vi "SplineHelp_getCubicSplinesFromControlVectors.vi"(9 "endCtrlVector":T3, 10 "InternalWaypoints":T4[](array[typedef]) {"Y" format="%14.3f"; "X" format="%14.3f"}, 11 "startCtrlVector":T3) -> (0 "error out":errorcluster, 3 "splines":T1[](array[typedef]), 4 "y final":dbl[][](array[numeric]), 5 "x final":dbl[][](array[numeric]), 6 "y init":dbl[][](array[numeric]), 7 "x init":dbl[][](array[numeric]))   [LabVIEW 2019, in "Trajectory_Library.lvlib"]
doc: "Returns a set of cubic splines corresponding to the provided control vectors. The user is free to set the direction of the start and end point. The directions for the middle waypoints are determined automatically to ensure continuous curvature throughout the path.\n\nParameters: \n - startCtrlVector - The starting control vector.\n - waypoints - The middle waypoints. This can be left blank if you only wish to create a path with two waypoints.\n - endCtrlVector - The ending control vector.\n\nReturns:\n - A vector of cubic hermite splines that interpolate through the provided waypoints and control vectors.\n - Error Out - Output error cluster\n - X init - For diagnostics only (these may be deleted in the future)\n - X final - For diagnostics only (these may be deleted in the future)\n - Y init - For diagnostics only (these may be deleted in the future)\n - Y final - For diagnostics only (these may be deleted in the future)"
uses:
  Trajectory_Library.lvlib
  SPLINE_CTRL_VECTOR.ctl
  TRANSLATION2D.ctl
  SPLINE.ctl
  <vilib>/Analysis/Matrix/Datatypes/RealMatrix.ctl
  <vilib>/Analysis/Matrix/NI_Matrix.lvlib
panel:
  # "for\ndebug!"
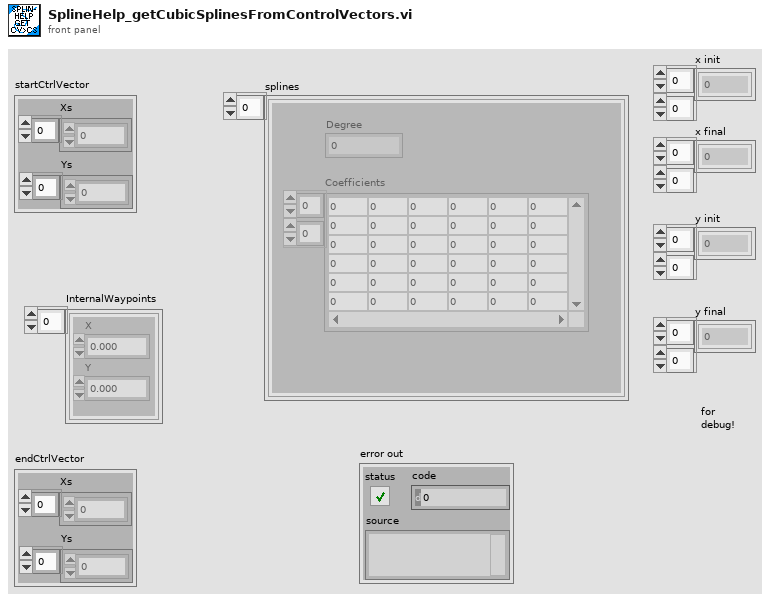
[diagram p1: front panel]
types:
  T1 = typedef "Trajectory_Library.lvlib/SPLINE.ctl" = cluster{"Degree":i32, "Coefficients":T2}
  T2 = typedef "NI_Matrix.lvlib/RealMatrix.ctl" = dbl[][]
  T3 = typedef "Trajectory_Library.lvlib/SPLINE_CTRL_VECTOR.ctl" = cluster{"Xs":dbl[], "Ys":dbl[]}
  T4 = typedef "Trajectory_Library.lvlib/TRANSLATION2D.ctl" = cluster{"X":dbl, "Y":dbl}
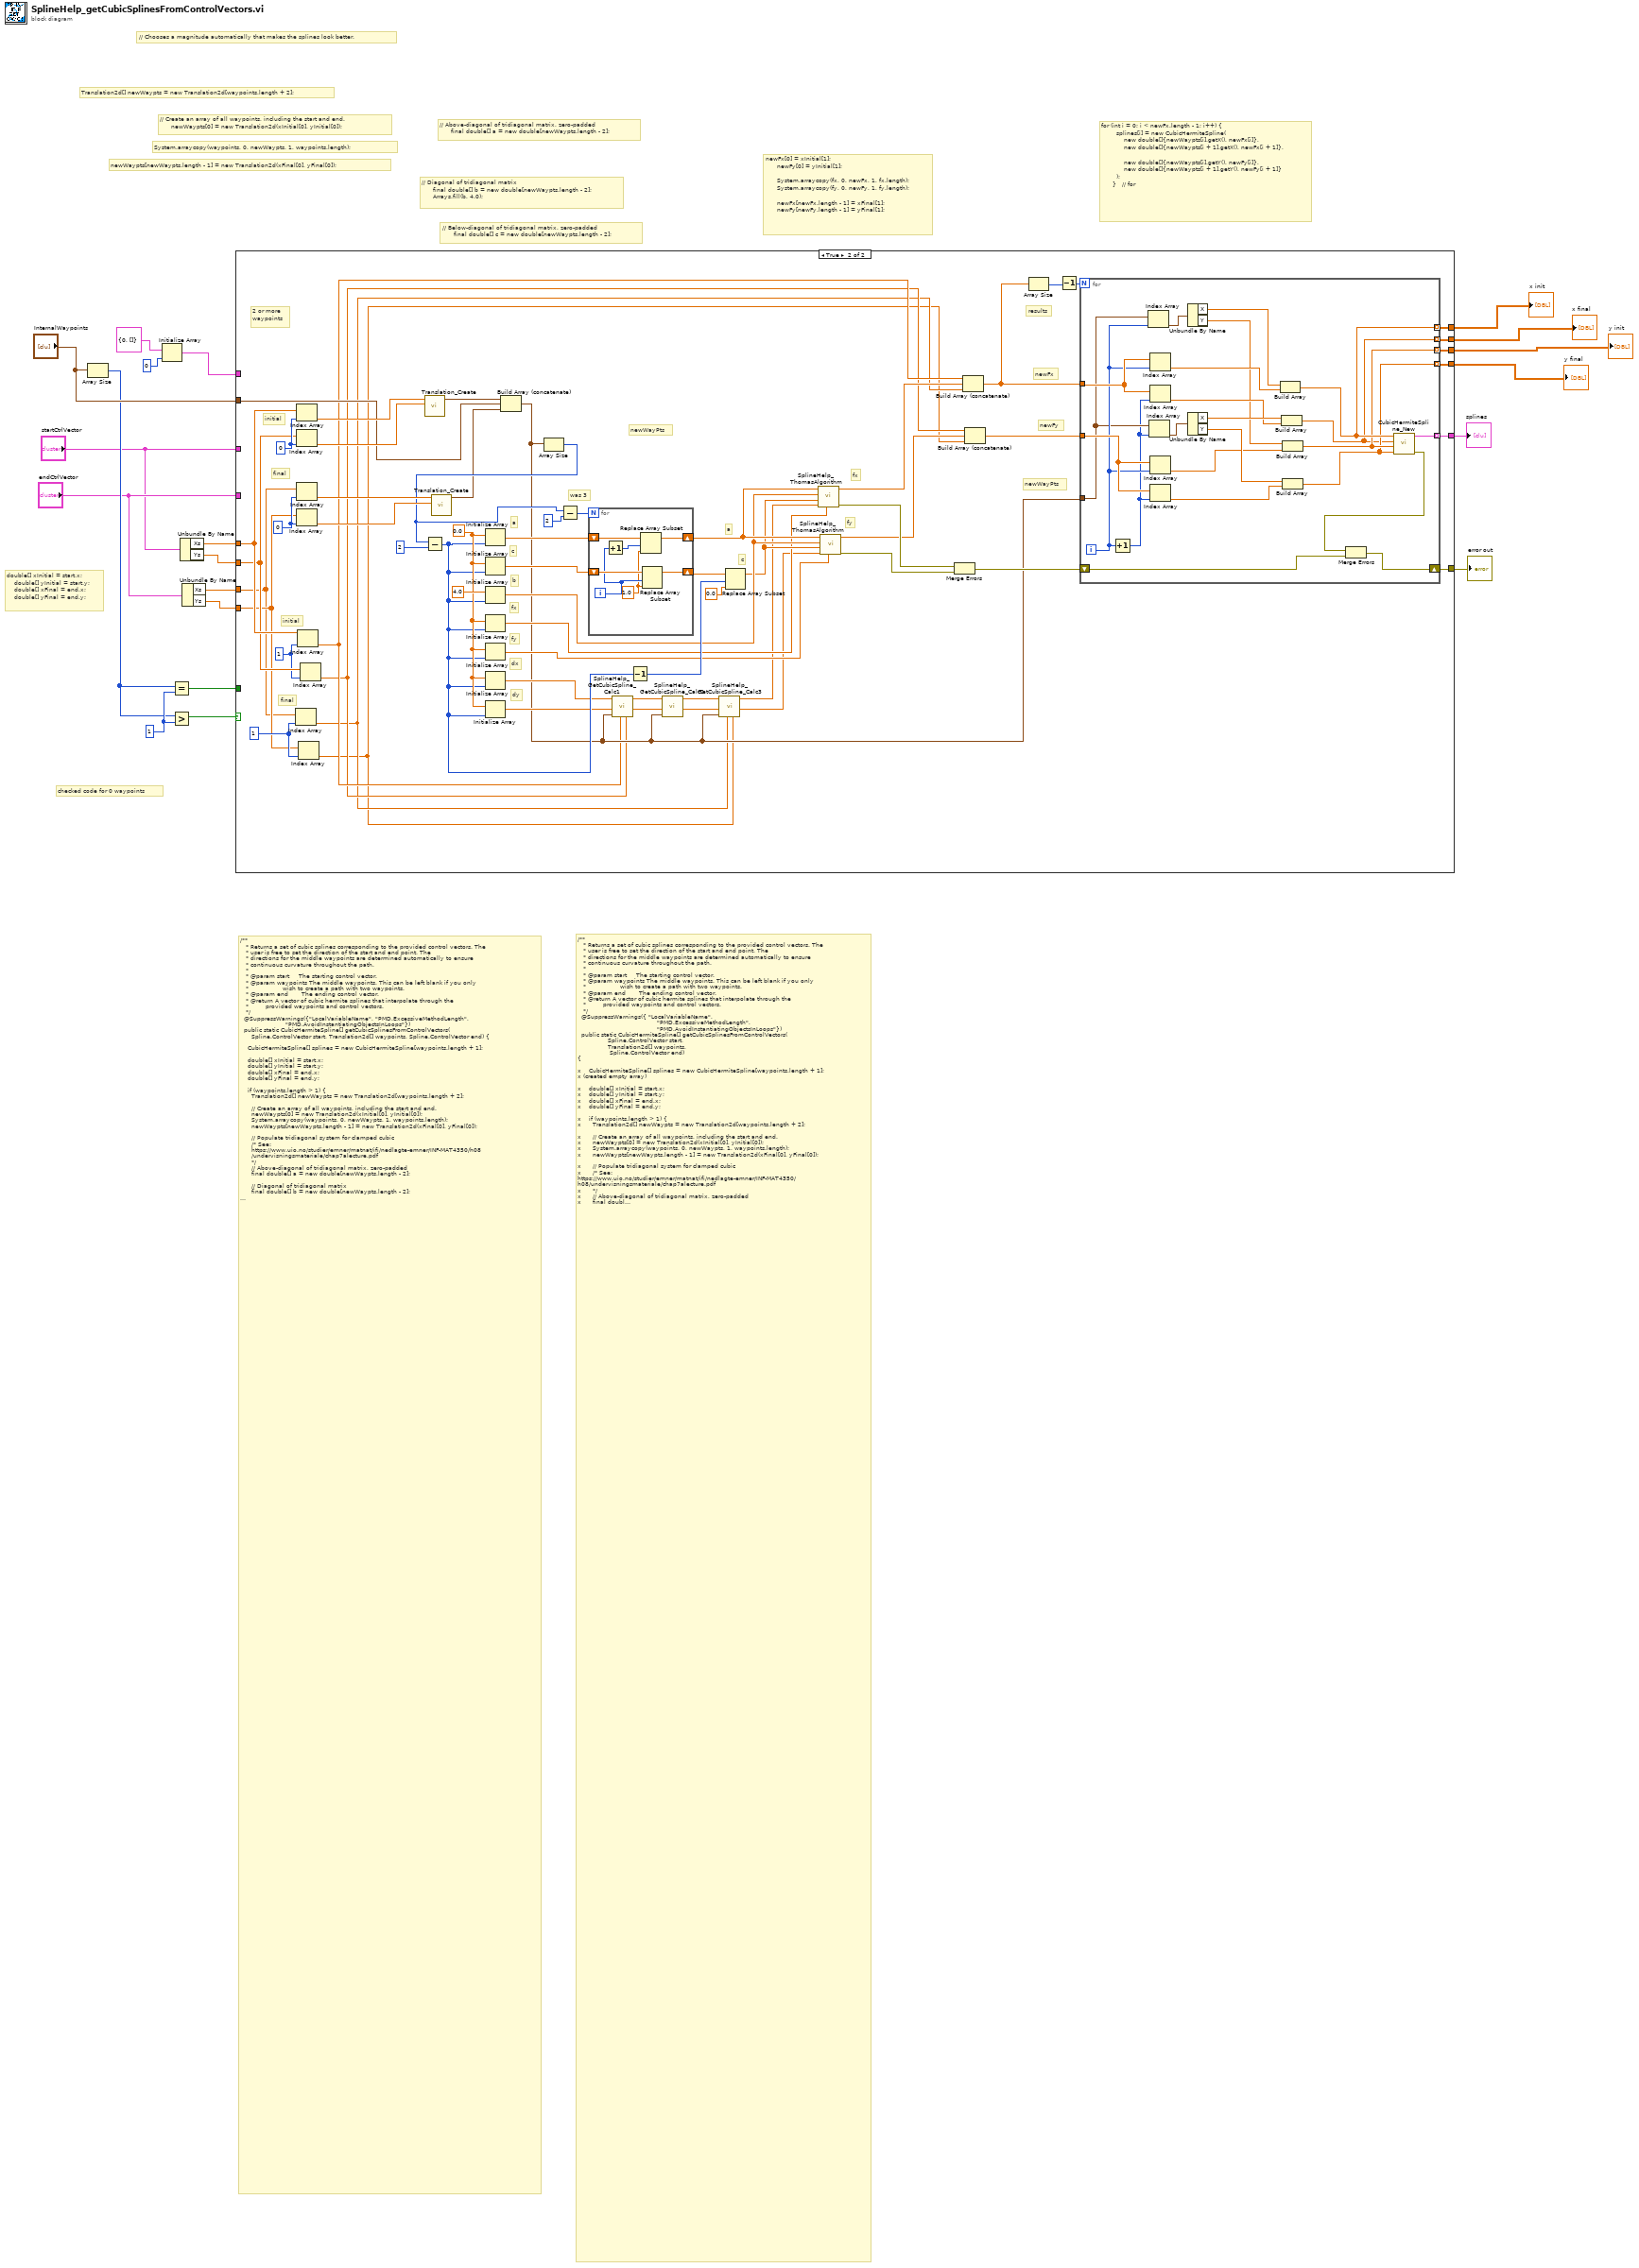
[diagram p0: block diagram]
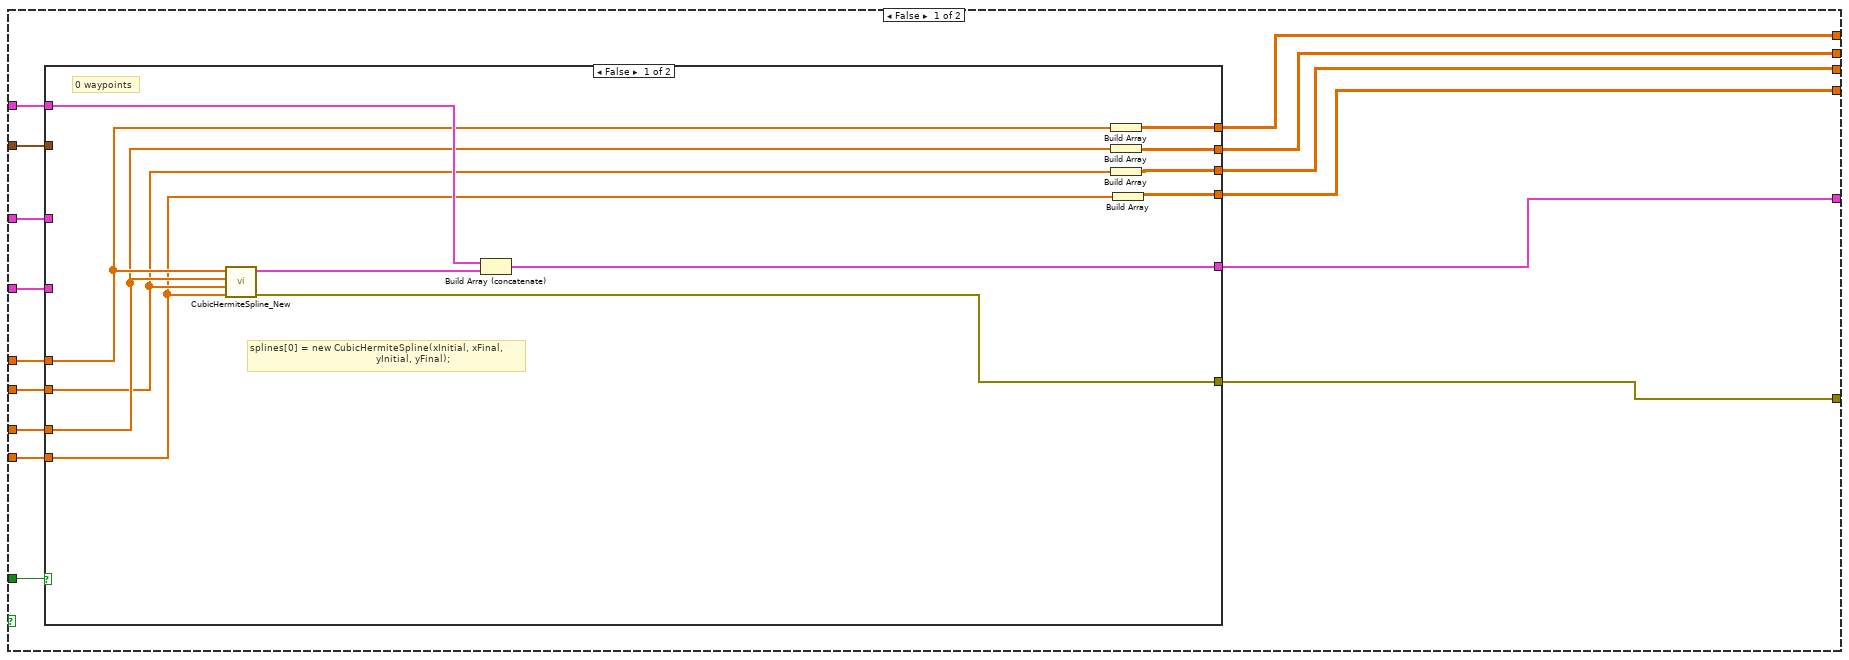
[diagram p2: hidden frame]
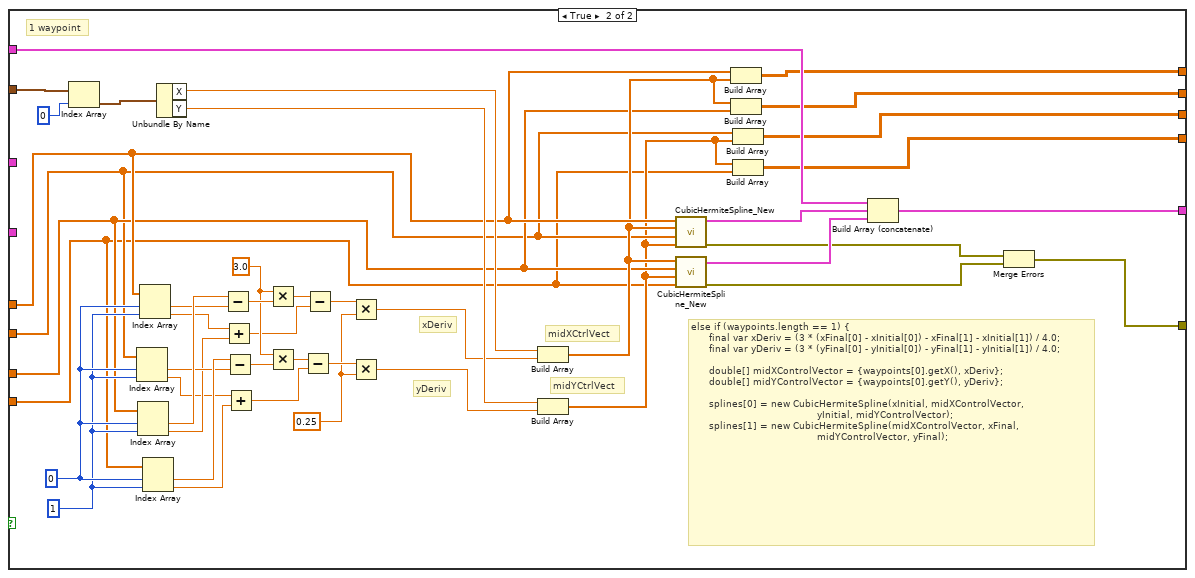
[diagram p3: hidden frame]
diagram:
  w18 = 1 ("y")
  # "for (int i = 0; i < newFx.length - 1; i++) {\n        splines[i] = new CubicHermiteSpline(\n            new double[]{newWaypts[i].getX(), newFx[i]},\n            new double[]{newWaypts[i + 1].getX(), newFx[i + 1]},\n\n            new double[]{newWaypts[i].getY(), newFy[i]},\n            new double[]{newWaypts[i + 1].getY(), newFy[i + 1]}\n        );\n      }   // for"
  # "/**\n   * Returns a set of cubic splines corresponding to the provided control vectors. The\n   * user is free to set the direction of the start and end point. The\n   * directions for the middle waypoints are determined automatically to ensure\n   * continuous curvature throughout the path.\n   *\n   * @param start     The starting control vector.\n   * @param waypoints The middle waypoints. This can be left blank if you only\n   *                  wish to create a path with two waypoints.\n   * @param end       The ending control vector.\n   * @return A vector of cubic hermite splines that interpolate through the\n   *         provided waypoints and control vectors.\n   */\n  @SuppressWarnings({ \"LocalVariableName\", \n                                          \"PMD.ExcessiveMethodLength\",\n                                          \"PMD.AvoidInstantiatingObjectsInLoops\"})\n  public static CubicHermiteSpline[] getCubicSplinesFromControlVectors(\n                Spline.ControlVector start, \n                Translation2d[] waypoints, \n                 Spline.ControlVector end) \n{\n\nx    CubicHermiteSpline[] splines = new CubicHermiteSpline[waypoints.length + 1];\nx (created empty array)\n\nx    double[] xInitial = start.x;\nx    double[] yInitial = start.y;\nx    double[] xFinal = end.x;\nx    double[] yFinal = end.y;\n\nx    if (waypoints.length > 1) {\nx      Translation2d[] newWaypts = new Translation2d[waypoints.length + 2];\n\nx      // Create an array of all waypoints, including the start and end.\nx      newWaypts[0] = new Translation2d(xInitial[0], yInitial[0]);\nx      System.arraycopy(waypoints, 0, newWaypts, 1, waypoints.length);\nx      newWaypts[newWaypts.length - 1] = new Translation2d(xFinal[0], yFinal[0]);\n\nx      // Populate tridiagonal system for clamped cubic\nx      /* See:      \nhttps://www.uio.no/studier/emner/matnat/ifi/nedlagte-emner/INF-MAT4350/\nh08/undervisningsmateriale/chap7alecture.pdf\nx      */\nx      // Above-diagonal of tridiagonal matrix, zero-padded\nx      final double[] a = new double[newWaypts.length - 2];\n\nx      // Diagonal of tridiagonal matrix\nx      final double[] b = new double[newWaypts.length - 2];\nx      Arrays.fill(b, 4.0);\n\nx      // Below-diagonal of tridiagonal matrix, zero-padded\nx      final double[] c = new double[newWaypts.length - 2];\n\nx      // rhs vectors\nx      final double[] dx = new double[newWaypts.length - 2];\nx      final double[] dy = new double[newWaypts.length - 2];\n\nx      // solution vectors\nx      final double[] fx = new double[newWaypts.length - 2];\nx      final double[] fy = new double[newWaypts.length - 2];\n\n      // populate above-diagonal and below-diagonal vectors\nx      a[0] = 0.0;\nx      for (int i = 0; i < newWaypts.length - 3; i++) {\nx        a[i + 1] = 1;\nx        c[i] = 1;\nx      }   //for\nx      c[c.length - 1] = 0.0;\n\nx SUBVI - CALC 1\nx      // populate rhs vectors\nx      dx[0] = 3 * (newWaypts[2].getX() - newWaypts[0].getX()) - xInitial[1];\nx      dy[0] = 3 * (newWaypts[2].getY() - newWaypts[0].getY()) - yInitial[1];\n\nx SUBVI - CALC 2\nx      if (newWaypts.length > 4)  { \nx        for (int i = 1; i <= newWaypts.length - 4; i++) {\nx          dx[i] = 3 * (newWaypts[i + 1].getX() - newWaypts[i - 1].getX());\nx          dy[i] = 3 * (newWaypts[i + 1].getY() - newWaypts[i - 1].getY());\nx        }  // for\nx      } // > 4\n\nx SUBVI - CALC 3\nx      dx[dx.length - 1] = 3 * (newWaypts[newWaypts.length - 1].getX()\nx          - newWaypts[newWaypts.length - 3].getX()) - xFinal[1];\nx      dy[dy.length - 1] = 3 * (newWaypts[newWaypts.length - 1].getY()\nx          - newWaypts[newWaypts.length - 3].getY()) - yFinal[1];\n\nx      // Compute solution to tridiagonal system\nx      thomasAlgorithm(a, b, c, dx, fx);\nx      thomasAlgorithm(a, b, c, dy, fy);\n\nx      double[] newFx = new double[fx.length + 2];\nx      double[] newFy = new double[fy.length + 2];\n\nx      newFx[0] = xInitial[1];\nx      newFy[0] = yInitial[1];\nx      System.arraycopy(fx, 0, newFx, 1, fx.length);\nx      System.arraycopy(fy, 0, newFy, 1, fy.length);\nx      newFx[newFx.length - 1] = xFinal[1];\nx      newFy[newFy.length - 1] = yFinal[1];\n\n      for (int i = 0; i < newFx.length - 1; i++) {\n        splines[i] = new CubicHermiteSpline(\n            new double[]{newWaypts[i].getX(), newFx[i]},\n            new double[]{newWaypts[i + 1].getX(), newFx[i + 1]},\n            new double[]{newWaypts[i].getY(), newFy[i]},\n            new double[]{newWaypts[i + 1].getY(), newFy[i + 1]}\n        );\n      }   // for\n    } else if (waypoints.length == 1) {\n      final var xDeriv = (3 * (xFinal[0]\n          - xInitial[0])\n          - xFinal[1] - xInitial[1])\n          / 4.0;\n      final var yDeriv = (3 * (yFinal[0]\n          - yInitial[0])\n          - yFinal[1] - yInitial[1])\n          / 4.0;\n\n      double[] midXControlVector = {waypoints[0].getX(), xDeriv};\n      double[] midYControlVector = {waypoints[0].getY(), yDeriv};\n\n      splines[0] = new CubicHermiteSpline(xInitial, midXControlVector,\n                                          yInitial, midYControlVector);\n      splines[1] = new CubicHermiteSpline(midXControlVector, xFinal,\n                                          midYControlVector, yFinal);\n    } else {\n      splines[0] = new CubicHermiteSpline(xInitial, xFinal,\n                                          yInitial, yFinal);\n    }\n    return splines;\n  }"
  # "// Below-diagonal of tridiagonal matrix, zero-padded\n      final double[] c = new double[newWaypts.length - 2];"
  # "// Diagonal of tridiagonal matrix\n      final double[] b = new double[newWaypts.length - 2];\n      Arrays.fill(b, 4.0);"
  # "// Above-diagonal of tridiagonal matrix, zero-padded\n      final double[] a = new double[newWaypts.length - 2];"
  # "newWaypts[newWaypts.length - 1] = new Translation2d(xFinal[0], yFinal[0]);"
  # "System.arraycopy(waypoints, 0, newWaypts, 1, waypoints.length);"
  # "// Create an array of all waypoints, including the start and end.\n      newWaypts[0] = new Translation2d(xInitial[0], yInitial[0]);"
  # "Translation2d[] newWaypts = new Translation2d[waypoints.length + 2];"
  # "checked code for 0 waypoints"
  # "double[] xInitial = start.x;\n    double[] yInitial = start.y;\n    double[] xFinal = end.x;\n    double[] yFinal = end.y;"
  # "newFx[0] = xInitial[1];\n      newFy[0] = yInitial[1];\n\n      System.arraycopy(fx, 0, newFx, 1, fx.length);\n      System.arraycopy(fy, 0, newFy, 1, fy.length);\n\n      newFx[newFx.length - 1] = xFinal[1];\n      newFy[newFy.length - 1] = yFinal[1];"
  # "/**\n   * Returns a set of cubic splines corresponding to the provided control vectors. The\n   * user is free to set the direction of the start and end point. The\n   * directions for the middle waypoints are determined automatically to ensure\n   * continuous curvature throughout the path.\n   *\n   * @param start     The starting control vector.\n   * @param waypoints The middle waypoints. This can be left blank if you only\n   *                  wish to create a path with two waypoints.\n   * @param end       The ending control vector.\n   * @return A vector of cubic hermite splines that interpolate through the\n   *         provided waypoints and control vectors.\n   */\n  @SuppressWarnings({\"LocalVariableName\", \"PMD.ExcessiveMethodLength\",\n                        \"PMD.AvoidInstantiatingObjectsInLoops\"})\n  public static CubicHermiteSpline[] getCubicSplinesFromControlVectors(\n      Spline.ControlVector start, Translation2d[] waypoints, Spline.ControlVector end) {\n\n    CubicHermiteSpline[] splines = new CubicHermiteSpline[waypoints.length + 1];\n\n    double[] xInitial = start.x;\n    double[] yInitial = start.y;\n    double[] xFinal = end.x;\n    double[] yFinal = end.y;\n\n    if (waypoints.length > 1) {\n      Translation2d[] newWaypts = new Translation2d[waypoints.length + 2];\n\n      // Create an array of all waypoints, including the start and end.\n      newWaypts[0] = new Translation2d(xInitial[0], yInitial[0]);\n      System.arraycopy(waypoints, 0, newWaypts, 1, waypoints.length);\n      newWaypts[newWaypts.length - 1] = new Translation2d(xFinal[0], yFinal[0]);\n\n      // Populate tridiagonal system for clamped cubic\n      /* See:\n      https://www.uio.no/studier/emner/matnat/ifi/nedlagte-emner/INF-MAT4350/h08\n      /undervisningsmateriale/chap7alecture.pdf\n      */\n      // Above-diagonal of tridiagonal matrix, zero-padded\n      final double[] a = new double[newWaypts.length - 2];\n\n      // Diagonal of tridiagonal matrix\n      final double[] b = new double[newWaypts.length - 2];\n      Arrays.fill(b, 4.0);\n\n      // Below-diagonal of tridiagonal matrix, zero-padded\n      final double[] c = new double[newWaypts.length - 2];\n\n      // rhs vectors\n      final double[] dx = new double[newWaypts.length - 2];\n      final double[] dy = new double[newWaypts.length - 2];\n\n      // solution vectors\n      final double[] fx = new double[newWaypts.length - 2];\n      final double[] fy = new double[newWaypts.length - 2];\n\n      // populate above-diagonal and below-diagonal vectors\n      a[0] = 0.0;\n      for (int i = 0; i < newWaypts.length - 3; i++) {\n        a[i + 1] = 1;\n        c[i] = 1;\n      }\n      c[c.length - 1] = 0.0;\n\n      // populate rhs vectors\n      dx[0] = 3 * (newWaypts[2].getX() - newWaypts[0].getX()) - xInitial[1];\n      dy[0] = 3 * (newWaypts[2].getY() - newWaypts[0].getY()) - yInitial[1];\n\n      if (newWaypts.length > 4) {\n        for (int i = 1; i <= newWaypts.length - 4; i++) {\n          dx[i] = 3 * (newWaypts[i + 1].getX() - newWaypts[i - 1].getX());\n          dy[i] = 3 * (newWaypts[i + 1].getY() - newWaypts[i - 1].getY());\n        }\n      }\n\n      dx[dx.length - 1] = 3 * (newWaypts[newWaypts.length - 1].getX()\n          - newWaypts[newWaypts.length - 3].getX()) - xFinal[1];\n      dy[dy.length - 1] = 3 * (newWaypts[newWaypts.length - 1].getY()\n          - newWaypts[newWaypts.length - 3].getY()) - yFinal[1];\n\n      // Compute solution to tridiagonal system\n      thomasAlgorithm(a, b, c, dx, fx);\n      thomasAlgorithm(a, b, c, dy, fy);\n\n      double[] newFx = new double[fx.length + 2];\n      double[] newFy = new double[fy.length + 2];\n\n      newFx[0] = xInitial[1];\n      newFy[0] = yInitial[1];\n      System.arraycopy(fx, 0, newFx, 1, fx.length);\n      System.arraycopy(fy, 0, newFy, 1, fy.length);\n      newFx[newFx.length - 1] = xFinal[1];\n      newFy[newFy.length - 1] = yFinal[1];\n\n      for (int i = 0; i < newFx.length - 1; i++) {\n        splines[i] = new CubicHermiteSpline(\n            new double[]{newWaypts[i].getX(), newFx[i]},\n            new double[]{newWaypts[i + 1].getX(), newFx[i + 1]},\n            new double[]{newWaypts[i].getY(), newFy[i]},\n            new double[]{newWaypts[i + 1].getY(), newFy[i + 1]}\n        );\n      }\n    } else if (waypoints.length == 1) {\n      final var xDeriv = (3 * (xFinal[0]\n          - xInitial[0])\n          - xFinal[1] - xInitial[1])\n          / 4.0;\n      final var yDeriv = (3 * (yFinal[0]\n          - yInitial[0])\n          - yFinal[1] - yInitial[1])\n          / 4.0;\n\n      double[] midXControlVector = {waypoints[0].getX(), xDeriv};\n      double[] midYControlVector = {waypoints[0].getY(), yDeriv};\n\n      splines[0] = new CubicHermiteSpline(xInitial, midXControlVector,\n                                          yInitial, midYControlVector);\n      splines[1] = new CubicHermiteSpline(midXControlVector, xFinal,\n                                          midYControlVector, yFinal);\n    } else {\n      splines[0] = new CubicHermiteSpline(xInitial, xFinal,\n                                          yInitial, yFinal);\n    }\n    return splines;\n  }"
  # "// Chooses a magnitude automatically that makes the splines look better."
  n1 = Array Size(array="InternalWaypoints") -> (size(s)=w12:i32)
  n2 = Initialize Array(T1 {"Degree"=0, "Coefficients"=[]} ("SPLINE"), 0 ("dimension size")) -> (w14:T1[])
  n3 = Equal?(x=w12, y=w18) -> (x = y?=w17:bool)
  n4 = Greater?(x=w12, y=w18) -> (0:w19:bool)
  n5 = Unbundle By Name("startCtrlVector") -> ("Xs"=w9:dbl[], "Ys"=w8:dbl[])
  n6 = Unbundle By Name("endCtrlVector") -> ("Xs"=w7:dbl[], "Ys"=w6:dbl[])
  n7 = case shown="True" w19 {
    tunnel: w17 -> [w35 _]
    tunnel: w14 -> [w34 _]
    tunnel: [w33 w130] -> w16
    tunnel: [w32 w123] -> w15
    tunnel: "startCtrlVector" -> [w31 _]
    tunnel: "endCtrlVector" -> [w30 _]
    tunnel: "InternalWaypoints" -> [w29 w106]
    tunnel: w9 -> [w28 w139]
    tunnel: w8 -> [w27 w138]
    tunnel: w7 -> [w26 w122]
    tunnel: w6 -> [w25 w128]
    tunnel: [w21 w95] -> w1
    tunnel: [w22 w94] -> w2
    tunnel: [w23 w93] -> w3
    tunnel: [w24 w92] -> w4
    frame False {
      n8 = case shown="False" w35 {
        tunnel: w34 -> [w47 w84]
        tunnel: [w46 w83] -> w33
        tunnel: [w44 w78] -> w32
        tunnel: w31 -> [_ _]
        tunnel: w30 -> [_ _]
        tunnel: w29 -> [_ w90]
        tunnel: w28 -> [w39 w57]
        tunnel: w27 -> [w37 w54]
        tunnel: w26 -> [w38 w55]
        tunnel: w25 -> [w36 w52]
        tunnel: [w43 w51] -> w24
        tunnel: [w42 w50] -> w23
        tunnel: [w41 w49] -> w22
        tunnel: [w40 w48] -> w21
        frame False {
          # "splines[0] = new CubicHermiteSpline(xInitial, xFinal,\n                                          yInitial, yFinal);"
          # "0 waypoints"
          n9 = call "CubicHermiteSpline_New.vi"("yFinalCtrlVector"=w36, "yInitialCtrlVector"=w37, "xFinalCtrlVector"=w38, "XInitialCtrlVector"=w39) -> ("error out"=w44:errorcluster, "CubicHermiteSpline"=w45:T1)  [unwired: 6 in]
          n10 = Build Array (concatenate)(w47, w45) -> (w46:T1[])
          n11 = Build Array(w39) -> (w43:dbl[][])
          n12 = Build Array(w38) -> (w42:dbl[][])
          n13 = Build Array(w37) -> (w41:dbl[][])
          n14 = Build Array(w36) -> (w40:dbl[][])
        }
        frame True {
          w60 = 0.25 ("y")
          w71 = 3.0 ("x")
          w85 = 1 ("index")
          w86 = 0 ("index")
          # "yDeriv"
          # "xDeriv"
          # "midYCtrlVect"
          # "midXCtrlVect"
          # "else if (waypoints.length == 1) {\n      final var xDeriv = (3 * (xFinal[0] - xInitial[0]) - xFinal[1] - xInitial[1]) / 4.0;\n      final var yDeriv = (3 * (yFinal[0] - yInitial[0]) - yFinal[1] - yInitial[1]) / 4.0;\n\n      double[] midXControlVector = {waypoints[0].getX(), xDeriv};\n      double[] midYControlVector = {waypoints[0].getY(), yDeriv};\n\n      splines[0] = new CubicHermiteSpline(xInitial, midXControlVector,\n                                          yInitial, midYControlVector);\n      splines[1] = new CubicHermiteSpline(midXControlVector, xFinal,\n                                          midYControlVector, yFinal);"
          # "1 waypoint"
          n15 = Index Array(array=w90, index=0) -> (element=w89:T4)
          n16 = Index Array(array=w54, index #1=w86, index #2=w85) -> (element #1=w74:dbl, element #2=w66:dbl)
          n17 = Index Array(array=w55, index #1=w86, index #2=w85) -> (element #1=w77:dbl, element #2=w70:dbl)
          n18 = Index Array(array=w57, index #1=w86, index #2=w85) -> (element #1=w76:dbl, element #2=w69:dbl)
          n19 = Index Array(array=w52, index #1=w86, index #2=w85) -> (element #1=w75:dbl, element #2=w65:dbl)
          n20 = Unbundle By Name(w89) -> ("X"=w88:dbl, "Y"=w87:dbl)
          n21 = Subtract(x=w77, y=w76) -> (x-y=w73:dbl)
          n22 = Add(x=w69, y=w70) -> (x+y=w67:dbl)
          n23 = Subtract(x=w75, y=w74) -> (x-y=w72:dbl)
          n24 = Add(x=w66, y=w65) -> (x+y=w63:dbl)
          n25 = Multiply(x=w71, y=w73) -> (x*y=w68:dbl)
          n26 = Multiply(x=w71, y=w72) -> (x*y=w64:dbl)
          n27 = Subtract(x=w64, y=w63) -> (x-y=w61:dbl)
          n28 = Subtract(x=w68, y=w67) -> (x-y=w62:dbl)
          n29 = Multiply(x=w62, y=w60) -> (x*y=w59:dbl)
          n30 = Multiply(x=w61, y=w60) -> (x*y=w58:dbl)
          n31 = Build Array(w88, w59) -> (w56:dbl[])
          n32 = Build Array(w87, w58) -> (w53:dbl[])
          n33 = call "CubicHermiteSpline_New.vi"("yFinalCtrlVector"=w53, "yInitialCtrlVector"=w54, "xFinalCtrlVector"=w56, "XInitialCtrlVector"=w57) -> ("error out"=w80:errorcluster, "CubicHermiteSpline"=w82:T1)  [unwired: 6 in]
          n34 = call "CubicHermiteSpline_New.vi"("yFinalCtrlVector"=w52, "yInitialCtrlVector"=w53, "xFinalCtrlVector"=w55, "XInitialCtrlVector"=w56) -> ("error out"=w79:errorcluster, "CubicHermiteSpline"=w81:T1)  [unwired: 6 in]
          n35 = Build Array(w57, w56) -> (w51:dbl[][])
          n36 = Build Array(w56, w55) -> (w50:dbl[][])
          n37 = Build Array(w54, w53) -> (w49:dbl[][])
          n38 = Build Array(w53, w52) -> (w48:dbl[][])
          n39 = Build Array (concatenate)(w84, w82, w81) -> (w83:T1[])
          n40 = Merge Errors(w80, w79) -> (w78:errorcluster)
        }
      }
    }
    frame True {
      w129 = 1 ("index")
      w137 = 1 ("index")
      w134 = 0.0
      w148 = 0 ("index")
      w151 = 0 ("index")
      # "was 3"
      # "newWayPts"
      # "newFy"
      # "newFx"
      # "2 or more\nwaypoints"
      # "results"
      # "initial"
      # "final"
      # "final"
      # "initial"
      # "fy"
      # "fx"
      # "c"
      # "a"
      # "dy"
      # "dx"
      # "fy"
      # "fx"
      # "b"
      # "c"
      # "a"
      # "newWayPts"
      n41 = Index Array(array=w122, index=w129) -> (element=w100:dbl)
      n42 = Index Array(array=w138, index=w151) -> (element=w149:dbl)
      n43 = Index Array(array=w128, index=w148) -> (element=w146:dbl)
      n44 = Index Array(array=w139, index=w151) -> (element=w150:dbl)
      n45 = Index Array(array=w122, index=w148) -> (element=w147:dbl)
      n46 = Index Array(array=w139, index=w137) -> (element=w102:dbl)
      n47 = Index Array(array=w128, index=w129) -> (element=w99:dbl)
      n48 = Index Array(array=w138, index=w137) -> (element=w101:dbl)
      n49 = call "Translation_Create.vi"("Y"=w149, "X"=w150) -> ("TRANSLATION"=w108:T4)  [unwired: 9 in]
      n50 = call "Translation_Create.vi"("Y"=w146, "X"=w147) -> ("TRANSLATION"=w107:T4)  [unwired: 9 in]
      n51 = Build Array (concatenate)(w108, w106, w107) -> (w105:T4[])
      n52 = Array Size(array=w105) -> (size(s)=w118:i32)
      n53 = Subtract(x=w118, y=2) -> (x-y=w117:i32)
      n54 = Initialize Array(w134, w117) -> (w145:dbl[])
      n55 = Initialize Array(w134, w117) -> (w136:dbl[])
      n56 = Initialize Array(4.0, w117) -> (w132:dbl[])
      n57 = Initialize Array(w134, w117) -> (w120:dbl[])
      n58 = Initialize Array(w134, w117) -> (w127:dbl[])
      n59 = Initialize Array(w134, w117) -> (w115:dbl[])
      n60 = Initialize Array(w134, w117) -> (w114:dbl[])
      n61 = Subtract(x=w118, y=2) -> (x-y=w144:i32)
      n62 = for {
        N: w144 -> [_]
        shift-right: [w175] -> w133
        shift-left: w145 -> [w181]
        shift-right: [w176] -> w141
        shift-left: w136 -> [w180]
        i -> [w178]
        w177 = 1.0 ("new element/subarray")
        n63 = Increment(x=w178) -> (x+1=w179:i32)
        n64 = Replace Array Subset(array=w181, new element=w177, index=w179) -> (w175:dbl[])
        n65 = Replace Array Subset(array=w180, new element=w177, index=w178) -> (w176:dbl[])
      }
      n66 = call "SplineHelp_GetCubicSpline_Calc1.vi"("Y-Initial-1"=w101, "X-Initial-1"=w102, "newWayPoints"=w105, "dy-in"=w114, "dx-in"=w115) -> ("dy-out"=w116:dbl[], "dx-out"=w112:dbl[])  [unwired: 5 in]
      n67 = Decrement(x=w117) -> (x-1=w140:i32)
      n68 = call "SplineHelp_GetCubicSpline_Calc2.vi"("newWayPts"=w105, "dy-in"=w116, "dx-in"=w112) -> ("dy-out"=w113:dbl[], "dx-out"=w109:dbl[])  [unwired: 7 in]
      n69 = call "SplineHelp_GetCubicSpline_Calc3.vi"("y-final-1"=w99, "x-final-1"=w100, "newWayPoints"=w105, "dy-in"=w113, "dx-in"=w109) -> ("dy-out"=w111:dbl[], "dx-out"=w110:dbl[])  [unwired: 5 in]
      n70 = Replace Array Subset(array=w141, new element=0.0 ("new element/subarray"), index=w140) -> (w131:dbl[])
      n71 = call "SplineHelp_ThomasAlgorithm.vi"("inputSolutionVector"=w120, "D"=w110, "C"=w131, "B"=w132, "A"=w133) -> ("error out"=w126:errorcluster, "SolutionVector"=w104:dbl[])  [unwired: 5 in]
      n72 = call "SplineHelp_ThomasAlgorithm.vi"("inputSolutionVector"=w127, "D"=w111, "C"=w131, "B"=w132, "A"=w133) -> ("error out"=w125:errorcluster, "SolutionVector"=w103:dbl[])  [unwired: 5 in]
      n73 = Merge Errors(w126, w125) -> (w124:errorcluster)
      n74 = Build Array (concatenate)(w102, w104, w100) -> (w96:dbl[])
      n75 = Build Array (concatenate)(w101, w103, w99) -> (w98:dbl[])
      n76 = Array Size(array=w96) -> (size(s)=w97:i32)
      n77 = Decrement(x=w97) -> (x-1=w119:i32)
      n78 = for {
        N: w119 -> [_]
        tunnel: [w174] -> w130 mode=indexing
        tunnel: w96 -> [w173]
        tunnel: w98 -> [w172]
        tunnel: w105 -> [w170]
        shift-right: [w157] -> w123
        shift-left: w124 -> [w158]
        tunnel: [w155] -> w92 mode=indexing
        tunnel: [w154] -> w94 mode=indexing
        tunnel: [w153] -> w95 mode=indexing
        tunnel: [w152] -> w93 mode=indexing
        i -> [w171]
        n79 = Increment(x=w171) -> (x+1=w169:i32)
        n80 = Index Array(array=w170, index=w171) -> (element=w168:T4)
        n81 = Index Array(array=w170, index=w169) -> (element=w167:T4)
        n82 = Index Array(array=w173, index=w171) -> (element=w165:dbl)
        n83 = Index Array(array=w173, index=w169) -> (element=w163:dbl)
        n84 = Index Array(array=w172, index=w171) -> (element=w160:dbl)
        n85 = Index Array(array=w172, index=w169) -> (element=w159:dbl)
        n86 = Unbundle By Name(w168) -> ("X"=w166:dbl, "Y"=w162:dbl)
        n87 = Unbundle By Name(w167) -> ("X"=w164:dbl, "Y"=w161:dbl)
        n88 = Build Array(w166, w165) -> (w155:dbl[])
        n89 = Build Array(w164, w163) -> (w152:dbl[])
        n90 = Build Array(w162, w160) -> (w154:dbl[])
        n91 = Build Array(w161, w159) -> (w153:dbl[])
        n92 = call "CubicHermiteSpline_New.vi"("yFinalCtrlVector"=w153, "yInitialCtrlVector"=w154, "xFinalCtrlVector"=w152, "XInitialCtrlVector"=w155) -> ("error out"=w156:errorcluster, "CubicHermiteSpline"=w174:T1)  [unwired: 6 in]
        n93 = Merge Errors(w156, w158) -> (w157:errorcluster)
      }
    }
  }
  "error out" <- w15
  "splines" <- w16
  "x init" <- w4
  "x final" <- w3
  "y init" <- w2
  "y final" <- w1
